vi "Set Cursor Position.vi"(8 "error in (no error)":errorcluster, 10 "Position":u8, 11 "Refnum in":T1) -> (0 "error out":errorcluster, 3 "Refnum out":T1)   [LabVIEW 2019, in "HD44780.lvlib"]
uses:
  HD44780.lvlib
  FPGA VI Reference.ctl
  <vilib>/Utility/error.llb/Error Cluster From Error Code.vi
  <vilib>/rvi/errors/niLvFpgaAdjustHostInterfaceError.vi
  <vilib>/rvi/interface/nirviReadWriteControl/nirviReadWriteControl.xnode
  NiFpgaLv.dll
  <vilib>/rvi/interface/Simulation/niFpgaSimulationCallBeginRW.vi
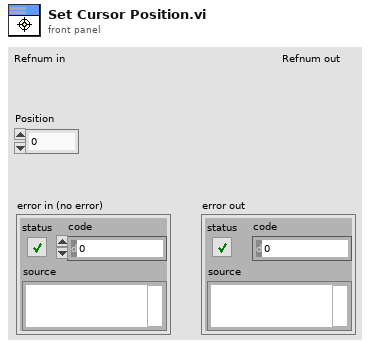
[diagram p1: front panel]
types:
  T1 = typedef "FPGA VI Reference.ctl" = refnum<k20>
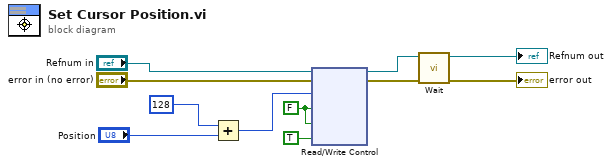
[diagram p0: block diagram]
diagram:
  w10 = FALSE ("RS")
  n1 = Add(x=u8 128, y="Position") -> (x+y=w5:u8)
  n2 = xnode "Read/Write Control"("FPGA VI Reference In"="Refnum in", "error in"="error in (no error)", "Data In"=w5, "RS"=w10, "R/W"=w10, "Enable"=TRUE) -> ("FPGA VI Reference Out"=w2:T1, "error out"=w4:errorcluster)
  n3 = call "Wait.vi"("error in (no error)"=w4, "Refnum in"=w2) -> ("error out"=→"error out":errorcluster, "Refnum out"=→"Refnum out":T1)  [unwired: 8 in]
